vi "Czas.vi"(7 "State":T1(ring), 8 "error in":errorcluster, 11 "Timer":dbl) -> (0 "error out":errorcluster, 1 "Time left":dbl, 2 "Elapsed Time":dbl, 3 "Time":bool, 5 "Pause":bool)   [LabVIEW 2020]
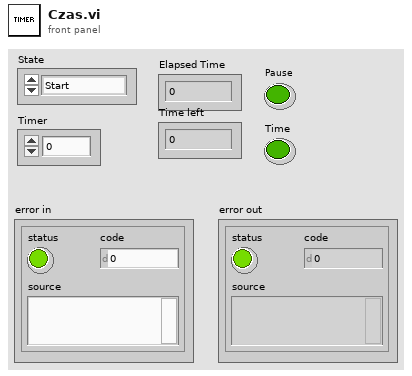
[diagram p1: front panel]
types:
  T1 = enum16{"Start", "Initialize", "Elapsed", "Pause"}
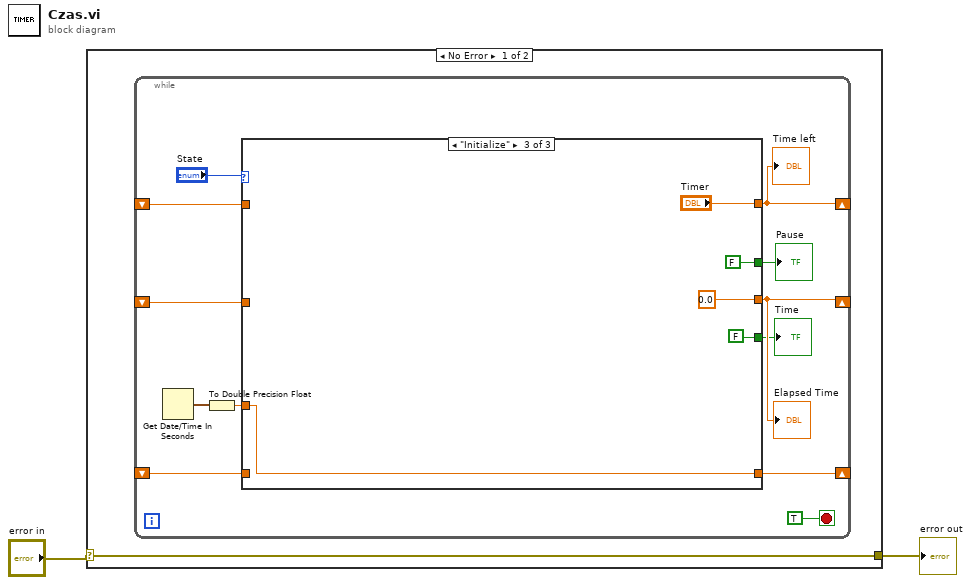
[diagram p0: block diagram]
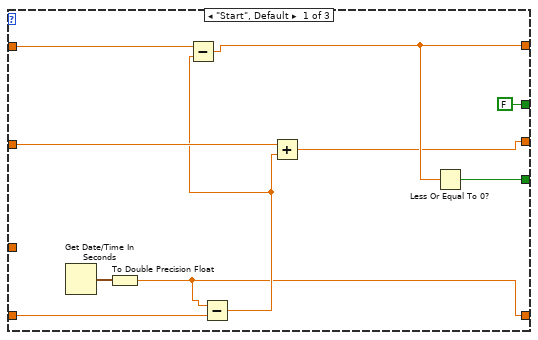
[diagram p2: hidden frame]
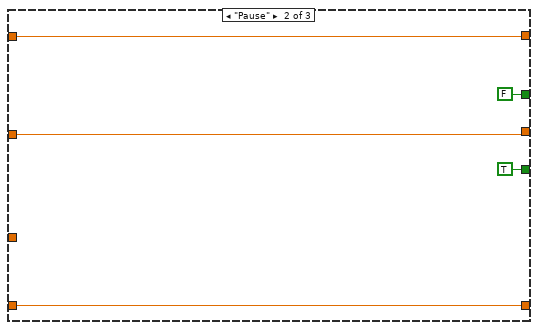
[diagram p3: hidden frame]
diagram:
  n1 = case shown="No Error" "error in" {
    selector: "error in" -> [w3 w36]
    tunnel: [w3 w36] -> w1
    frame No Error {
      n2 = while {
        shift-right: [w14] -> _
        shift-left: _ -> [w7]
        shift-right: [w13] -> _
        shift-left: _ -> [w6]
        shift-right: [w8] -> _
        shift-left: _ -> [w5]
        stop <- TRUE stop-if-true
        n3 = Get Date/Time In Seconds() -> (seconds since 1Jan1904=w10:timestamp)
        n4 = To Double Precision Float(number=w10) -> (double precision float=w9:dbl)
        n5 = case shown="\"Initialize\"" "State" {
          tunnel: [w22 w30 "Timer"] -> w14
          tunnel: [w20 w27 0.0] -> w13
          tunnel: [FALSE ("Pause") FALSE ("Pause") FALSE ("Pause")] -> w12
          tunnel: [w23 TRUE ("Pause") FALSE ("Pause")] -> w11
          tunnel: w9 -> [_ _ w31]
          tunnel: [w17 w26 w31] -> w8
          tunnel: w7 -> [w24 w30 _]
          tunnel: w6 -> [w21 w27 _]
          tunnel: w5 -> [w19 w26 _]
          frame "Start", Default {
            n6 = Get Date/Time In Seconds() -> (seconds since 1Jan1904=w25:timestamp)
            n7 = To Double Precision Float(number=w25) -> (double precision float=w17:dbl)
            n8 = Subtract(x=w17, y=w19) -> (x-y=w18:dbl)
            n9 = Subtract(x=w24, y=w18) -> (x-y=w22:dbl)
            n10 = Add(x=w21, y=w18) -> (x+y=w20:dbl)
            n11 = Less Or Equal To 0?(x=w22) -> (x <= 0?=w23:bool)
          }
          frame "Pause" {
          }
          frame "Initialize" {
          }
        }
        "Pause" <- w12
        "Time" <- w11
        "Elapsed Time" <- w13
        "Time left" <- w14
      }
    }
    frame Error {
    }
  }
  "error out" <- w1
